vi "Control.vi"(8 "error in (no error)":errorcluster, 11 "Logger in.lvclass":refnum<class "Logger.lvclass">) -> (0 "error out":errorcluster, 1 "tag count":i32, 2 "Start":bool, 3 "Logger out.lvclass":refnum<class "Logger.lvclass">, 4 "tag publish interval":i32, 5 "tag updates":i32)   [LabVIEW 2017, in "Logger.lvclass"]
uses:
  Logger.lvclass
  Logger.lvclass/Logger.ctl
  <vilib>/Skyline/Message/AMQP/NI Skyline Message AMQP (Sync).lvclass
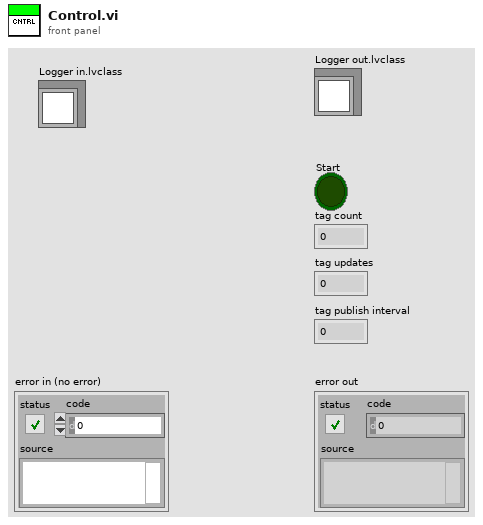
[diagram p1: front panel]
types:
  T1 = cluster{"tag_updates":i32, "tag_publish_interval":i32, "tag_count":i32}
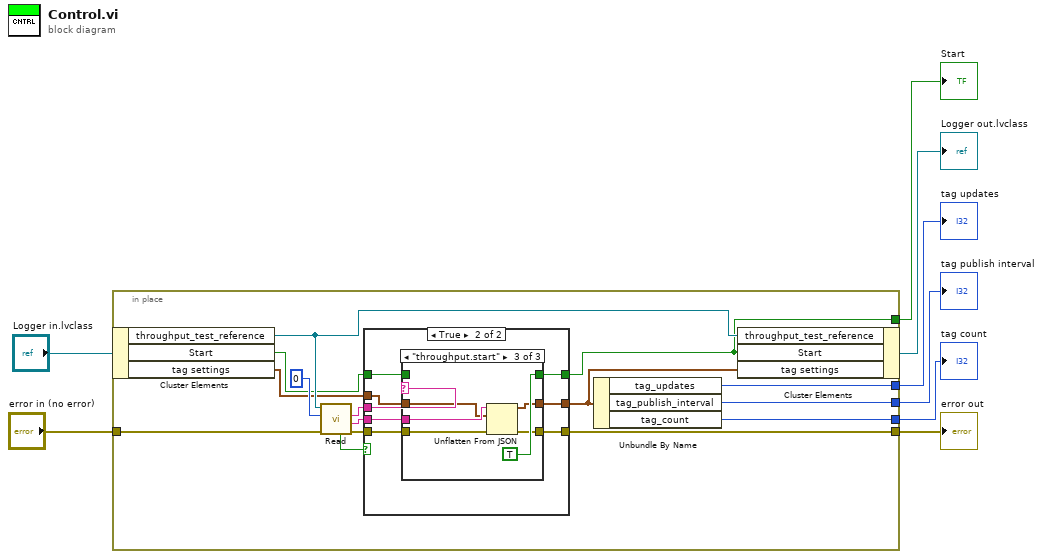
[diagram p0: block diagram]
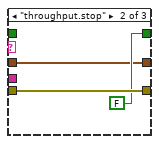
[diagram p4: hidden frame]
diagram:
  n1 = in-place {
    in-place-border: [w23] -> w5
    in-place-border: "error in (no error)" -> [w21]
    in-place-border: [w17] -> w6
    in-place-border: [w11] -> w3
    in-place-border: [w10] -> w2
    in-place-border: [w9] -> w1
    n2 = in-place-cluster #1("Logger in.lvclass") -> ("throughput_test_reference"=w19:refnum<class "NI Skyline Message AMQP (Sync).lvclass">, "Start"=w16:bool, "tag settings"=w13:T1)
    n3 = call-dynamic "Read.vi"("error in (no error)"=w21, "timeout milliseconds (100)"=0 ("timeout milliseconds"), "message sync"=w19) -> ("error out"=w22:errorcluster, "message"=w14:string, "topic"=w15:string, "dequeue status"=w18:bool)  [unwired: 4 in, 1 out]
    n4 = case shown="True" w18 {
      tunnel: w22 -> [w26 w32]
      tunnel: [w26 w31] -> w23
      tunnel: [w25 w34] -> w17
      tunnel: w16 -> [w25 w33]
      tunnel: w15 -> [_ w30]
      tunnel: w14 -> [_ w29]
      tunnel: w13 -> [w24 w28]
      tunnel: [w24 w27] -> w12
      frame False {
      }
      frame True {
        n5 = case shown="\"throughput.start\"" w30 {
          tunnel: [w37 FALSE ("Start") TRUE ("Start")] -> w34
          tunnel: w33 -> [w37 _ _]
          tunnel: w32 -> [w36 w40 w44]
          tunnel: [w36 w40 w41] -> w31
          tunnel: w29 -> [_ _ w45]
          tunnel: w28 -> [w35 w38 w43]
          tunnel: [w35 w38 w42] -> w27
          frame Default {
          }
          frame "throughput.stop" {
          }
          frame "throughput.start" {
            n6 = Unflatten From JSON(JSON string=w45, type and defaults=w43, error in (no error)=w44) -> (value=w42:T1, error out=w41:errorcluster)  [unwired: 4 in]
          }
        }
      }
    }
    n7 = Unbundle By Name(w12) -> ("tag_updates"=w11:i32, "tag_publish_interval"=w10:i32, "tag_count"=w9:i32)
    n8 = in-place-cluster #1("throughput_test_reference"=w19, "Start"=w17, "tag settings"=w12) -> (→"Logger out.lvclass":refnum<class "Logger.lvclass">)
  }
  "error out" <- w5
  "Start" <- w6
  "tag publish interval" <- w2
  "tag count" <- w1
  "tag updates" <- w3
